vi "Get Error Bar XY.vi"(4 "Marker Size":dbl, 6 "Base":dbl[](array[numeric]), 7 "Error Y?":bool=TRUE, 8 "error in (no error)":errorcluster, 9 "Min":dbl[](array[numeric]), 10 "Max":dbl[](array[numeric]), 11 "Plot Area Ref":refnum<vi>) -> (0 "error out":errorcluster, 2 "Error Bar XY":cluster{"X":i16, "X":i16}[][](array[cluster]), 3 "Dup Plot Area Ref":refnum<vi>)   [LabVIEW 2017, in "2D Error Bar.lvclass"]
uses:
  <vilib>/Math Plots/2D Math Plots/2D Error Bar/2D Error Bar/2D Error Bar.lvclass
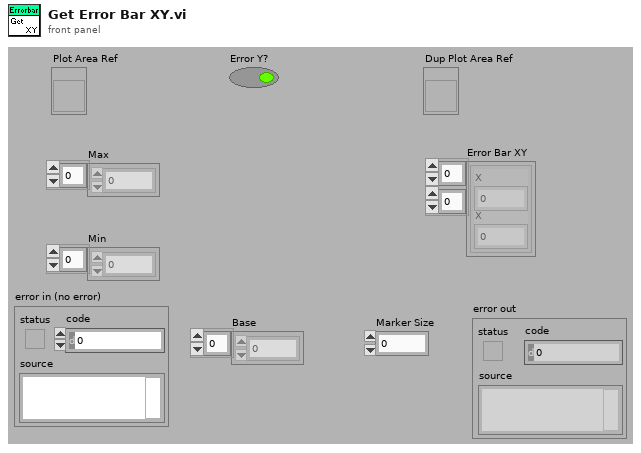
[diagram p1: front panel]
types:
  T1 = typedef "LVPoint32TypeDef.ctl" = cluster{"Horizontal":i32, "Vertical":i32}
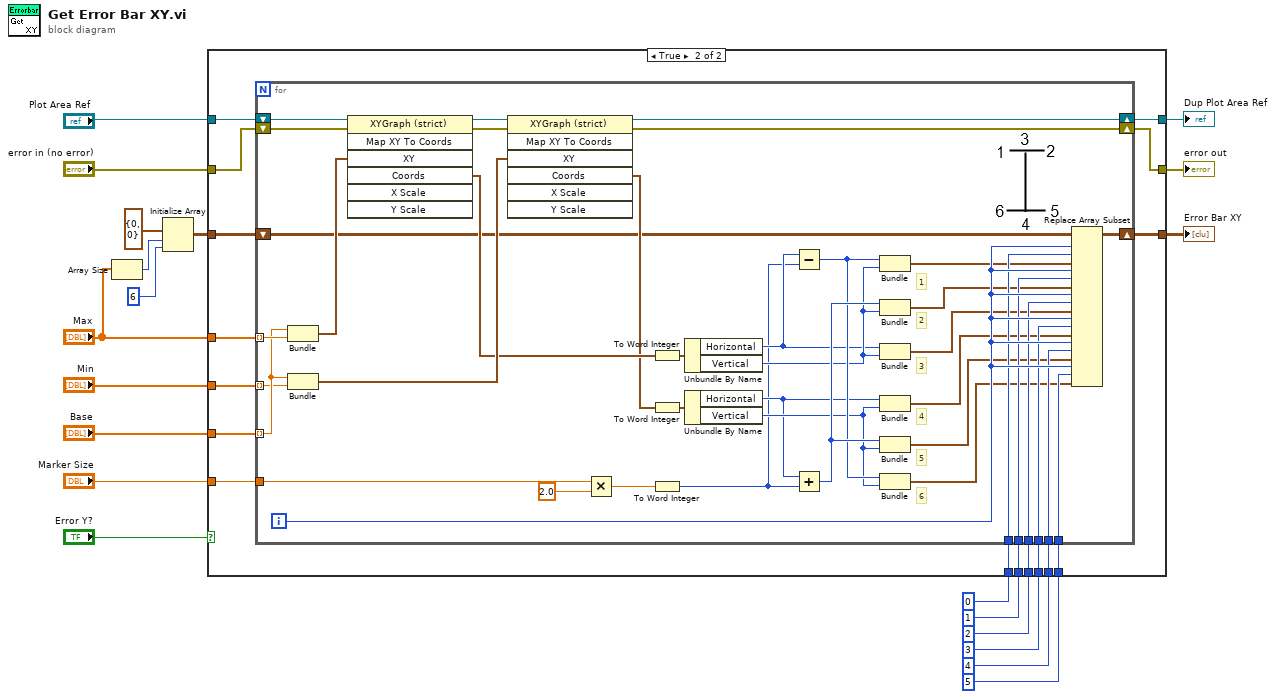
[diagram p0: block diagram]
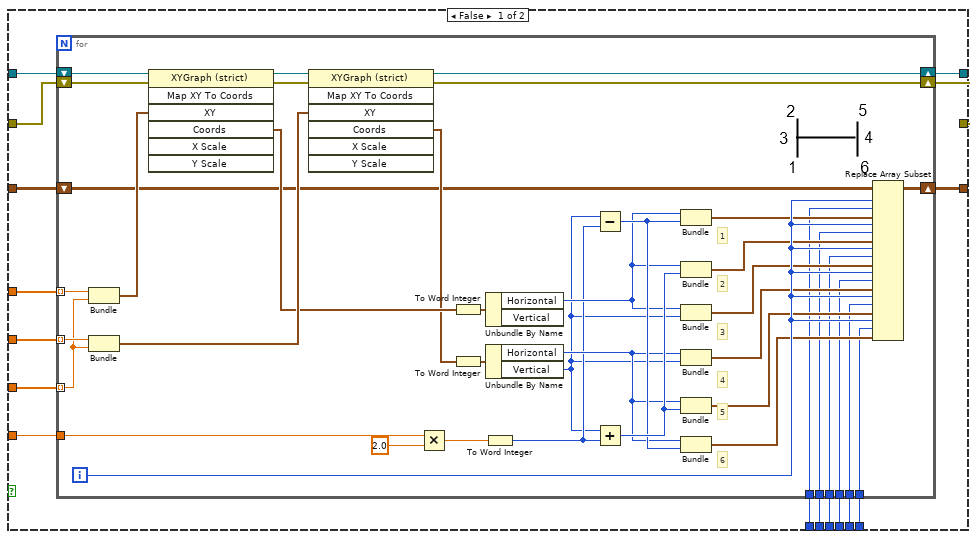
[diagram p2: hidden frame]
diagram:
  n1 = Array Size(array="Max") -> (size(s)=w7:i32)
  n2 = Initialize Array(cluster{"X":i16, "Y":i16} {"X"=0, "Y"=0} ("XY"), w7, 6 ("dimension size")) -> (w8:cluster{"X":i16, "Y":i16}[][])
  n3 = case shown="True" "Error Y?" {
    tunnel: "Max" -> [w36 w91]
    tunnel: "Min" -> [w35 w90]
    tunnel: [w27 w82] -> w19
    tunnel: "Marker Size" -> [w33 w89]
    tunnel: "Base" -> [w34 w88]
    tunnel: "Plot Area Ref" -> [w32 w87]
    tunnel: "error in (no error)" -> [w31 w86]
    tunnel: [w29 w85] -> w13
    tunnel: [w30 w84] -> w12
    tunnel: w8 -> [w28 w83]
    tunnel: 0 -> [w26 w81]
    tunnel: 1 -> [w25 w80]
    tunnel: 2 -> [w24 w79]
    tunnel: 3 -> [w23 w78]
    tunnel: 4 -> [w22 w77]
    tunnel: 5 -> [w21 w76]
    frame False {
      n4 = for {
        tunnel: w36 -> [w60] mode=indexing
        tunnel: w35 -> [w59] mode=indexing
        tunnel: w34 -> [w58] mode=indexing
        tunnel: w33 -> [w74]
        shift-right: [w53] -> w30
        shift-left: w32 -> [w62]
        shift-right: [w54] -> w29
        shift-left: w31 -> [w61]
        shift-right: [w51] -> w27
        shift-left: w28 -> [w50]
        tunnel: w26 -> [w42]
        tunnel: w25 -> [w41]
        tunnel: w24 -> [w40]
        tunnel: w23 -> [w39]
        tunnel: w22 -> [w38]
        tunnel: w21 -> [w37]
        i -> [w49]
        # "6"
        # "5"
        # "4"
        # "3"
        # "2"
        # "1"
        n5 = Bundle("X"=w60, "X"=w58) -> (w70:cluster{"X":dbl, "X":dbl})  [unwired: 1 out]
        n6 = Bundle("X"=w59, "X"=w58) -> (w67:cluster{"X":dbl, "X":dbl})  [unwired: 1 out]
        n7 = invoke class="XYGraph (strict)" method="Map XY To Coords"(reference=w62, error in=w61, "XY"=w70) -> (reference out=w69:refnum<vi>, error out=w68:errorcluster, "Coords"=w66:T1)  [unwired: 4 in, 4 out]
        n8 = invoke class="XYGraph (strict)" method="Map XY To Coords"(reference=w69, error in=w68, "XY"=w67) -> (reference out=w53:refnum<vi>, error out=w54:errorcluster, "Coords"=w65:T1)  [unwired: 4 in, 4 out]
        n9 = Multiply(x=w74, y=2.0) -> (x*y=w73:dbl)
        n10 = To Word Integer(number=w66) -> (16bit integer=w64:cluster{"Horizontal":i16, "Vertical":i16})
        n11 = To Word Integer(number=w65) -> (16bit integer=w63:cluster{"Horizontal":i16, "Vertical":i16})
        n12 = To Word Integer(number=w73) -> (16bit integer=w55:i16)
        n13 = Unbundle By Name(w64) -> ("Horizontal"=w57:i16)  [unwired: 1 out]
        n14 = Unbundle By Name(w63) -> ("Horizontal"=w56:i16, "Vertical"=w52:i16)
        n15 = Subtract(x=w52, y=w55) -> (x-y=w71:i16)
        n16 = Add(x=w52, y=w55) -> (x+y=w72:i16)
        n17 = Bundle("Horizontal"=w57, w71) -> (w48:cluster{"Horizontal":i16, i16})  [unwired: 1 out]
        n18 = Bundle("Horizontal"=w57, w72) -> (w47:cluster{"Horizontal":i16, i16})  [unwired: 1 out]
        n19 = Bundle("Horizontal"=w57, "Vertical"=w52) -> (w46:cluster{"Horizontal":i16, "Vertical":i16})  [unwired: 1 out]
        n20 = Bundle("Horizontal"=w56, "Vertical"=w52) -> (w45:cluster{"Horizontal":i16, "Vertical":i16})  [unwired: 1 out]
        n21 = Bundle("Horizontal"=w56, w72) -> (w44:cluster{"Horizontal":i16, i16})  [unwired: 1 out]
        n22 = Bundle("Horizontal"=w56, w71) -> (w43:cluster{"Horizontal":i16, i16})  [unwired: 1 out]
        n23 = Replace Array Subset(array=w50, new element #1=w48, index (row) #1=w49, index (col) #1=w42, new element #2=w47, index (row) #2=w49, index (col) #2=w41, new element #3=w46, index (row) #3=w49, index (col) #3=w40, new element #4=w45, index (row) #4=w49, index (col) #4=w39, new element #5=w44, index (row) #5=w49, index (col) #5=w38, new element #6=w43, index (row) #6=w49, index (col) #6=w37) -> (w51:cluster{"X":i16, "Y":i16}[][])
      }
    }
    frame True {
      n24 = for {
        tunnel: w91 -> [w129] mode=indexing
        tunnel: w90 -> [w124] mode=indexing
        tunnel: w88 -> [w125] mode=indexing
        tunnel: w89 -> [w110]
        shift-right: [w119] -> w84
        shift-left: w87 -> [w122]
        shift-right: [w113] -> w85
        shift-left: w86 -> [w114]
        shift-right: [w105] -> w82
        shift-left: w83 -> [w106]
        tunnel: w81 -> [w103]
        tunnel: w80 -> [w102]
        tunnel: w79 -> [w101]
        tunnel: w78 -> [w100]
        tunnel: w77 -> [w99]
        tunnel: w76 -> [w98]
        i -> [w104]
        # "6"
        # "5"
        # "4"
        # "3"
        # "2"
        # "1"
        n25 = Bundle("X"=w125, "X"=w129) -> (w128:cluster{"X":dbl, "X":dbl})  [unwired: 1 out]
        n26 = Bundle("X"=w125, "X"=w124) -> (w123:cluster{"X":dbl, "X":dbl})  [unwired: 1 out]
        n27 = invoke class="XYGraph (strict)" method="Map XY To Coords"(reference=w122, error in=w114, "XY"=w128) -> (reference out=w127:refnum<vi>, error out=w126:errorcluster, "Coords"=w121:T1)  [unwired: 4 in, 4 out]
        n28 = invoke class="XYGraph (strict)" method="Map XY To Coords"(reference=w127, error in=w126, "XY"=w123) -> (reference out=w119:refnum<vi>, error out=w113:errorcluster, "Coords"=w120:T1)  [unwired: 4 in, 4 out]
        n29 = Multiply(x=w110, y=2.0) -> (x*y=w109:dbl)
        n30 = To Word Integer(number=w121) -> (16bit integer=w112:cluster{"Horizontal":i16, "Vertical":i16})
        n31 = To Word Integer(number=w120) -> (16bit integer=w111:cluster{"Horizontal":i16, "Vertical":i16})
        n32 = To Word Integer(number=w109) -> (16bit integer=w107:i16)
        n33 = Unbundle By Name(w112) -> ("Horizontal"=w115:i16, "Vertical"=w118:i16)
        n34 = Unbundle By Name(w111) -> ("Horizontal"=w116:i16, "Vertical"=w117:i16)
        n35 = Subtract(x=w115, y=w107) -> (x-y=w130:i16)
        n36 = Add(x=w116, y=w107) -> (x+y=w131:i16)
        n37 = Bundle(w130, "Vertical"=w118) -> (w97:cluster{i16, "Vertical":i16})  [unwired: 1 out]
        n38 = Bundle(w131, "Vertical"=w118) -> (w96:cluster{i16, "Vertical":i16})  [unwired: 1 out]
        n39 = Bundle("Horizontal"=w115, "Vertical"=w118) -> (w95:cluster{"Horizontal":i16, "Vertical":i16})  [unwired: 1 out]
        n40 = Bundle("Horizontal"=w116, "Vertical"=w117) -> (w94:cluster{"Horizontal":i16, "Vertical":i16})  [unwired: 1 out]
        n41 = Bundle(w131, "Vertical"=w117) -> (w93:cluster{i16, "Vertical":i16})  [unwired: 1 out]
        n42 = Bundle(w130, "Vertical"=w117) -> (w92:cluster{i16, "Vertical":i16})  [unwired: 1 out]
        n43 = Replace Array Subset(array=w106, new element #1=w97, index (row) #1=w104, index (col) #1=w103, new element #2=w96, index (row) #2=w104, index (col) #2=w102, new element #3=w95, index (row) #3=w104, index (col) #3=w101, new element #4=w94, index (row) #4=w104, index (col) #4=w100, new element #5=w93, index (row) #5=w104, index (col) #5=w99, new element #6=w92, index (row) #6=w104, index (col) #6=w98) -> (w105:cluster{"X":i16, "Y":i16}[][])
      }
    }
  }
  "Error Bar XY" <- w19
  "Dup Plot Area Ref" <- w12
  "error out" <- w13
